vi "Soros port olvasás ver 3.0.vi"() -> ()   [LabVIEW 2020]
uses:
  <vilib>/Instr/_visa.llb/VISA Configure Serial Port (Instr).vi
  <vilib>/Utility/file.llb/Write Delimited Spreadsheet (string).vi
panel:
  in  "CSV Fájl kimentése":path
  out "Aktuális idõ":string
  out "Mozgásérzékelõ":bool
  out "Feszültségérték:":string
  in  "Port Kiválasztása":refnum<visa-resource-name>
  in  "Stop Button":bool
  # "V"
  # "Kommunikácós portok"
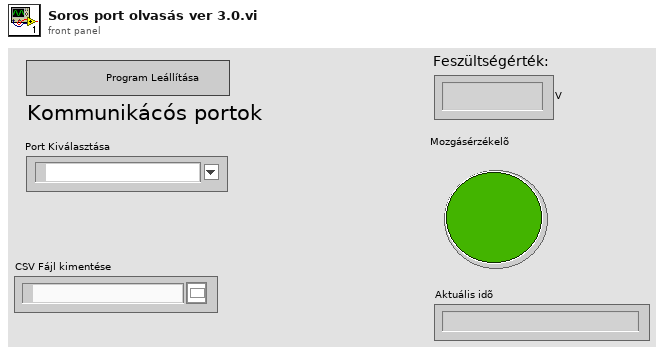
[diagram p1: front panel]
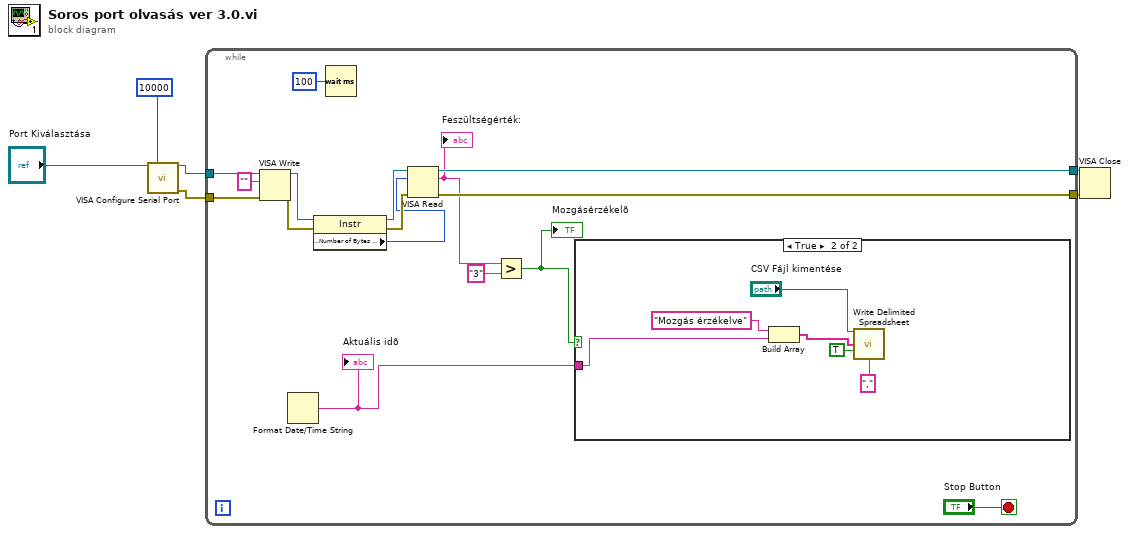
[diagram p0: block diagram]
diagram:
  n1 = call-poly "VISA Configure Serial Port"("VISA resource name"="Port Kiválasztása", "timeout (10sec)"=u32 10000) -> ("VISA resource name out"=w5:refnum<visa-resource-name>, "error out"=w3:errorcluster)  [unwired: 12 in]
  n2 = while {
    tunnel: w5 -> [w22]
    tunnel: [w21] -> w4
    tunnel: w3 -> [w20]
    tunnel: [w19] -> w2
    stop <- "Stop Button" stop-if-true
    n3 = VISA Write(VISA resource name=w22, write buffer="", error in (no error)=w20) -> (VISA resource name out=w18:refnum<visa-resource-name>, error out=w16:errorcluster)  [unwired: 1 out]
    n4 = Format Date/Time String() -> (date/time string=w7:string)  [unwired: 3 in]
    "Aktuális idõ" <- w7
    n5 = property class="Instr"(reference=w18, error in=w16) -> (reference out=w17:refnum<visa-resource-name>, error out=w15:errorcluster, "Serial Settings:Number of Bytes at Serial Port"=w14:u32)
    n6 = Wait (ms)(milliseconds to wait=u32 100) -> ()  [unwired: 1 out]
    n7 = VISA Read(VISA resource name=w17, byte count=w14, error in (no error)=w15) -> (VISA resource name out=w21:refnum<visa-resource-name>, read buffer=w9:string, error out=w19:errorcluster)  [unwired: 1 out]
    "Feszültségérték:" <- w9
    n8 = Greater?(x=w9, y="3") -> (0:w8:bool)
    "Mozgásérzékelõ" <- w8
    n9 = case shown="True" w8 {
      tunnel: w7 -> [_ w25]
      frame False {
      }
      frame True {
        n10 = Build Array("Mozgás érzékelve", w25) -> (w24:string[])
        n11 = call-poly <vilib>:"Write Delimited Spreadsheet.vi"("file path (dialog if empty)"="CSV Fájl kimentése", "1D data"=w24, "append to file? (new file:F)"=TRUE, "delimiter (\\t)"="," ("delimiter (\\t)")) -> ()  [unwired: 10 in, 2 out]
      }
    }
  }
  n12 = VISA Close(VISA resource name=w4, error in (no error)=w2) -> ()  [unwired: 1 out]
